vi "ReadGyro.vi"(5 "Teleop Local Data":T1 {"Vision"."Theta_Y" format="%.1f"; "Vision"."Theta_X" format="%.1f"; "Potentio" format="%.1f"; "Drive_Enc_R" format="%.1f"; "Drive_Enc_L" format="%.1f"; "Gyro_Angle" format="%.1f"; "Encoder_Lift" format="%.1f"; "Motor_Lift" format="%.3f"; "Motor_Intake" format="%.3f"; "Drive_Twist" format="%.3f"; "Drive_Forward" format="%.3f"}, 9 "error in":errorcluster) -> (6 "Out Teleop Local Data":T1 {"Vision"."Theta_Y" format="%.1f"; "Vision"."Theta_X" format="%.1f"; "Potentio" format="%.1f"; "Drive_Enc_R" format="%.1f"; "Drive_Enc_L" format="%.1f"; "Gyro_Angle" format="%.1f"; "Encoder_Lift" format="%.1f"; "Motor_Lift" format="%.3f"; "Motor_Intake" format="%.3f"; "Drive_Twist" format="%.3f"; "Drive_Forward" format="%.3f"}, 10 "error out":errorcluster)   [LabVIEW 2018]
uses:
  Typedefs/typedef_cluster_TeleOp_Local_Data.ctl
  Typedefs/typedef_cluster_Joystick.ctl
  Typedefs/typedef_cluster_Vision.ctl
  Typedefs/typedef_enum_refnums.ctl
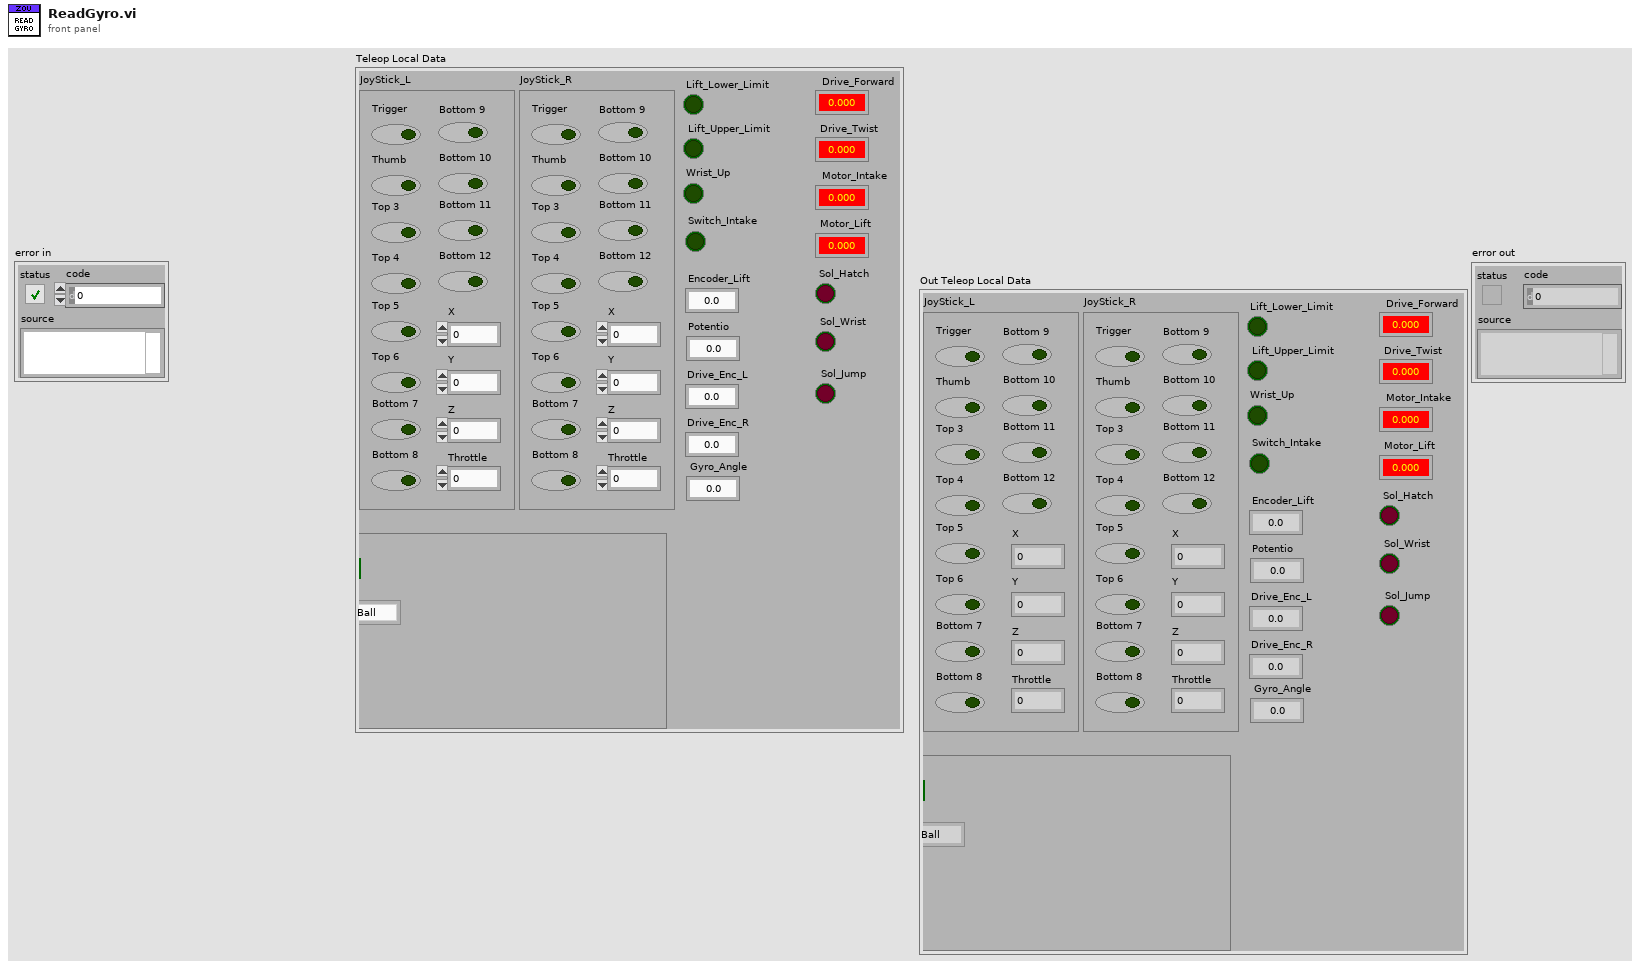
[diagram p1: front panel]
types:
  T1 = typedef "typedef_cluster_TeleOp_Local_Data.ctl" = cluster{"Lift_Lower_Limit":bool, "Wrist_Up":bool, "Switch_Intake":bool, "Encoder_Lift":dbl, "Sol_Wrist":bool, "Motor_Intake":dbl, "Motor_Lift":dbl, "Drive_Forward":dbl, "Drive_Twist":dbl, "Sol_Hatch":bool, "Gyro_Angle":dbl, "Drive_Enc_L":dbl, "Drive_Enc_R":dbl, "JoyStick_L":T2, "JoyStick_R":T2, "Potentio":dbl, "Vision":T3, "Lift_Upper_Limit":bool, "Sol_Jump":bool}
  T2 = typedef "typedef_cluster_Joystick.ctl" = cluster{"X":dbl, "Y":dbl, "Z":dbl, "Throttle":dbl, "Trigger":bool, "Thumb":bool, "Top 3":bool, "Top 4":bool, "Top 5":bool, "Top 6":bool, "Bottom 7":bool, "Bottom 8":bool, "Bottom 9":bool, "Bottom 10":bool, "Bottom 11":bool, "Bottom 12":bool}
  T3 = typedef "typedef_cluster_Vision.ctl" = cluster{"Theta_X":dbl, "Theta_Y":dbl, "Has_Target":bool, "Seek_Ball":bool, "Pipeline":enum16{"Ball", "Dual_Target", "Single_Target"}}
  T4 = typedef "typedef_enum_refnums.ctl" = enum16{"Joy_L", "Joy_R", "Drive_Motors", "Intake_Motor", "Wrist_Solenoid", "Hatch_Solenoid", "Compressor", "Lift_Motor", "Lift_Motor_2", "Gyro", "Drive_Enc_L", "Drive_Enc_R", "Lift_Lower_Limit", "Lift_Upper_Limit", "Ball_Switch", "Jump_Solenoid"}
  T5 = typedef "WPI_GyroDevRef.ctl" = cluster{"DevStatus":errorcluster, "Analog Channel":T6, "Gain (VoltsPerDegree/Second)":dbl, "Gyro Type":enum16{"Analog", "XRS450"}, "Handle":i32, "SPI Bus":T7, "Device Found":bool, "Sample Rate":dbl, "Calibrate On Open":bool, "Offset":dbl}
  T6 = typedef "FPGA_AIChannel.ctl" = enum8{"AI 0", "AI 1", "AI 2", "AI 3", "AI MXP 0", "AI MXP 1", "AI MXP 2", "AI MXP 3", "Invalid"}
  T7 = typedef "spi_bus.ctl" = enum16{"SPI On-Board, CS0", "SPI On-Board, CS1", "SPI On-Board, CS2", "SPI On-Board, CS3", "SPI MXP", "Invalid"}
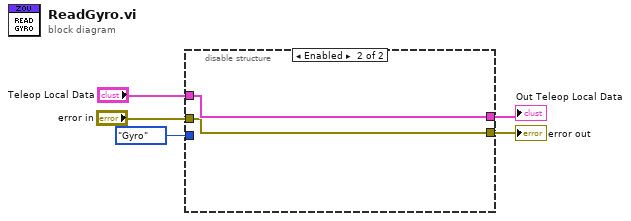
[diagram p0: block diagram]
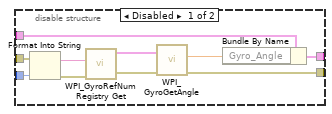
[diagram p2: hidden frame]
diagram:
  n1 = disable-structure shown="Enabled" {
    disable-tunnel: [w15 w17] -> w5
    disable-tunnel: "Teleop Local Data" -> [w14 w17]
    disable-tunnel: typedef_enum_refnums."Gyro" ("Enum") -> [w8 _]
    disable-tunnel: "error in" -> [w7 w16]
    disable-tunnel: [w6 w16] -> w1
    frame Disabled {
      n2 = Format Into String(error in=w7, w8) -> (resulting string=w12:string, error out=w9:errorcluster)  [unwired: 2 in]
      n3 = call <vilib>:"WPI_GyroRefNum Registry Get.vi"("error in (no error)"=w9, "refnum name"=w12) -> ("error out"=w10:errorcluster, "GyroDevRef"=w11:T5)  [unwired: 8 in]
      n4 = call <vilib>:"WPI_GyroGetAngle.vi"("error in"=w10, "GyroDevRef"=w11) -> ("error out"=w6:errorcluster, "Angle"=w13:dbl)  [unwired: 5 in, 3 out]
      n5 = Bundle By Name(cluster=w14, "Gyro_Angle"=w13) -> (w15:T1)
    }
    frame Enabled {
    }
  }
  "Out Teleop Local Data" <- w5
  "error out" <- w1
